vi "get_node_indicies.vi"(9 "File":string="SensorLocations.csv", 11 "Calibrations":string="Calibrations") -> (3 "Sensor Indicies":i32[](array[numeric]))   [LabVIEW 2018]
uses:
  <vilib>/Utility/file.llb/Read Delimited Spreadsheet (I64).vi
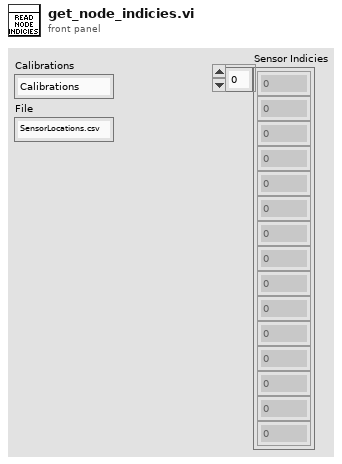
[diagram p1: front panel]
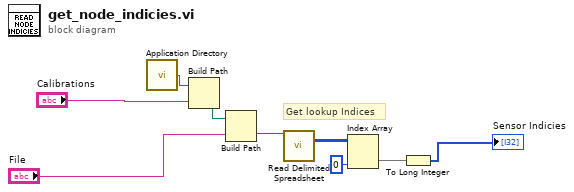
[diagram p0: block diagram]
diagram:
  # "Get lookup Indices"
  n1 = call <vilib>:"Application Directory.vi"() -> ("Application Directory"=w2:path)
  n2 = Build Path(base path=w2, name or relative path="Calibrations") -> (appended path=w3:path)
  n3 = Build Path(base path=w3, name or relative path="File") -> (appended path=w1:path)
  n4 = call-poly <vilib>:"Read Delimited Spreadsheet.vi"("file path (dialog if empty)"=w1) -> ("all rows"=w5:i64[][])  [unwired: 9 in, 5 out]
  n5 = Index Array(array=w5, index (col)=0 ("disabled index (col)")) -> (element=w4:i64[])  [unwired: 1 in]
  n6 = To Long Integer(number=w4) -> (32bit integer=→"Sensor Indicies":i32[])
